vi "GetBounds.vi"(8 "error in (no error)":errorcluster, 11 "separator item in":refnum<class "separator item.lvclass">) -> (0 "error out":errorcluster, 2 "bounds":cluster{"width":u32, "height":u32}, 3 "separator item out":refnum<class "separator item.lvclass">)   [LabVIEW 2009, in "separator item.lvclass"]
uses:
  separator item.lvclass
  separator item.lvclass/separator item.ctl
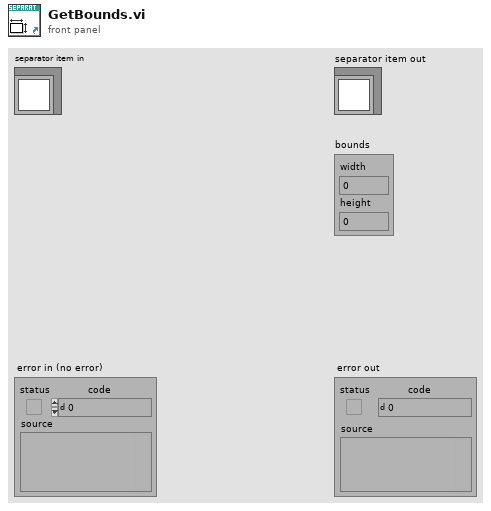
[diagram p1: front panel]
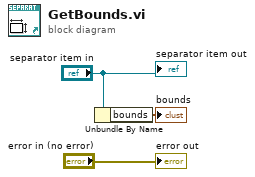
[diagram p0: block diagram]
diagram:
  n1 = Unbundle By Name("separator item in") -> ("bounds"=→"bounds":cluster{"width":u32, "height":u32})
  "error out" <- "error in (no error)"
  "separator item out" <- "separator item in"
